vi "SetRange.vi"(7 "Enum":enum16{"Auto Range", "10V and 10GOm"}(ring), 8 "error in":errorcluster, 11 "instrument handle in":refnum<k15>) -> (0 "error out":errorcluster, 3 "instrument handle out":refnum<k15>)   [LabVIEW 2017]
uses:
  <instrlib>/niDMM/nidmm.llb/niDMM Resolution in Digits.ctl
  <instrlib>/niDMM/nidmm.llb/niDMM Function.ctl
  <instrlib>/niDMM/nidmm.llb/niDMM Configure Measurement Digits.vi
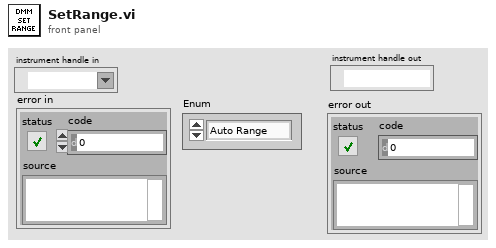
[diagram p1: front panel]
types:
  T1 = typedef "niDMM Function.ctl" = enum16{"DC Volts", "AC Volts", "DC Current", "AC Current", "2-wire Resistance", "4-wire Resistance", "Diode", "Frequency", "Period", "AC Volts DC Coupled", "Capacitance", "Inductance", "Temperature"}
  T2 = typedef "niDMM Resolution in Digits.ctl" = dbl
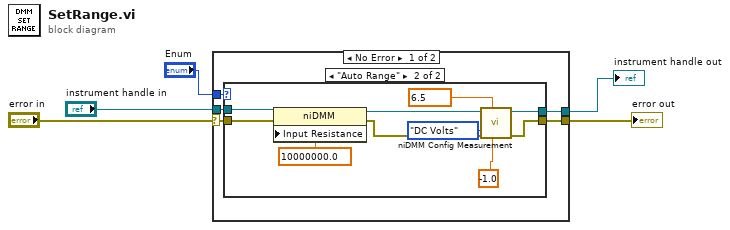
[diagram p0: block diagram]
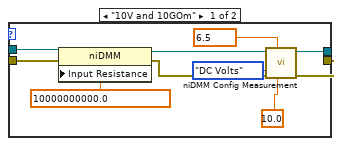
[diagram p2: hidden frame]
diagram:
  n1 = case shown="No Error" "error in" {
    selector: "error in" -> [w9 w31]
    tunnel: "instrument handle in" -> [w10 w32]
    tunnel: [w8 w32] -> w2
    tunnel: [w7 w31] -> w1
    tunnel: "Enum" -> [w6 _]
    frame No Error {
      n2 = case shown="\"Auto Range\"" w6 {
        tunnel: w10 -> [w20 w30]
        tunnel: w9 -> [w13 w23]
        tunnel: [w12 w22] -> w8
        tunnel: [w11 w21] -> w7
        frame "10V and 10GOm" {
          w17 = T2 6.5 items=["3 1/2"=3.5, "4 1/2"=4.5, "5 1/2"=5.5, "6 1/2"=6.5, "7 1/2"=7.5] ("Resolution in Digits")
          w19 = 10000000000.0 items=["1 M Ohm"=1000000.0, "10 M Ohm"=10000000.0, "Greater Than 10 G Ohm"=10000000000.0] ("Configuration:Measurement Options:Input Resistance")
          n3 = property class="niDMM"(reference=w20, error in=w13, "Input Resistance"=w19) -> (reference out=w15:refnum<k15>, error out=w14:errorcluster)
          n4 = call-poly <instrlib>:"niDMM Config Measurement.vi"("Range"=10.0, "Resolution in Digits"=w17, "error in (no error)"=w14, "Function"=niDMM_Function."DC Volts", "instrument handle"=w15) -> ("error out"=w11:errorcluster, "instrument handle out"=w12:refnum<k15>)  [unwired: 5 in]
        }
        frame "Auto Range" {
          w27 = T2 6.5 items=["3 1/2"=3.5, "4 1/2"=4.5, "5 1/2"=5.5, "6 1/2"=6.5, "7 1/2"=7.5] ("Resolution in Digits")
          w29 = 10000000.0 items=["1 M Ohm"=1000000.0, "10 M Ohm"=10000000.0, "Greater Than 10 G Ohm"=10000000000.0] ("Configuration:Measurement Options:Input Resistance")
          n5 = property class="niDMM"(reference=w30, error in=w23, "Input Resistance"=w29) -> (reference out=w25:refnum<k15>, error out=w24:errorcluster)
          n6 = call-poly <instrlib>:"niDMM Config Measurement.vi"("Range"=-1.0, "Resolution in Digits"=w27, "error in (no error)"=w24, "Function"=niDMM_Function."DC Volts", "instrument handle"=w25) -> ("error out"=w21:errorcluster, "instrument handle out"=w22:refnum<k15>)  [unwired: 5 in]
        }
      }
    }
    frame Error {
    }
  }
  "instrument handle out" <- w2
  "error out" <- w1
